vi "CV curve generator.vi"(0 "Lower bound (V)":dbl, 5 "Upper bound (V)":dbl, 7 "Start potential (V)":dbl, 9 "Stop potential (V)":dbl, 11 "Scan rate (mV/s)":dbl, 12 "Time (ms)":dbl, 13 "Number of cycles":u16) -> (4 "Actual potential":dbl, 15 "End":bool)   [LabVIEW 2015]
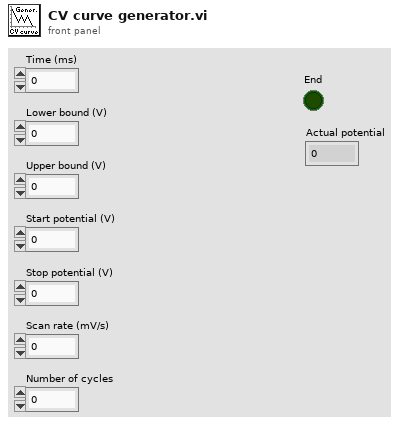
[diagram p1: front panel]
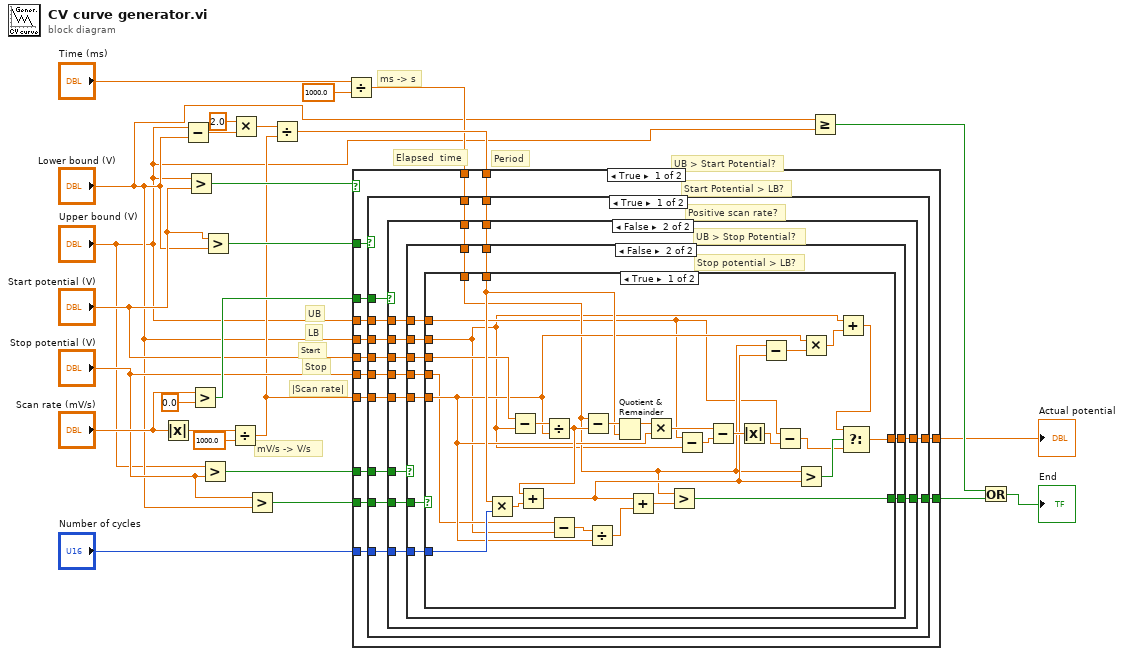
[diagram p0: block diagram]
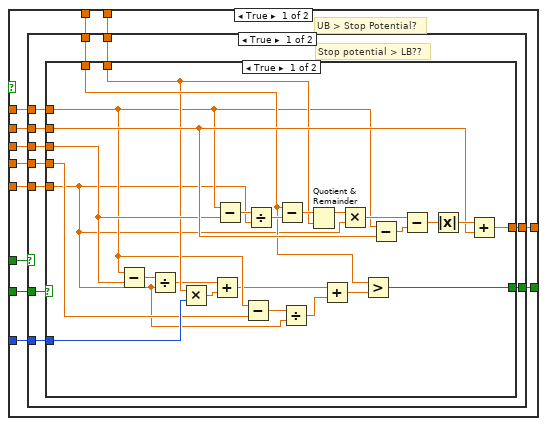
[diagram p2: hidden frame]
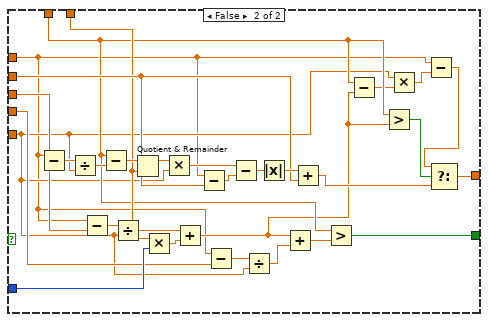
[diagram p3: hidden frame]
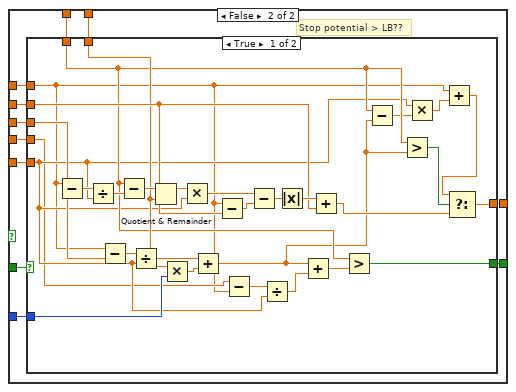
[diagram p4: hidden frame]
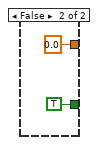
[diagram p5: hidden frame]
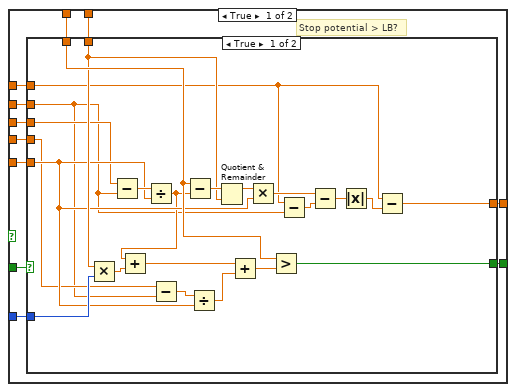
[diagram p6: hidden frame]
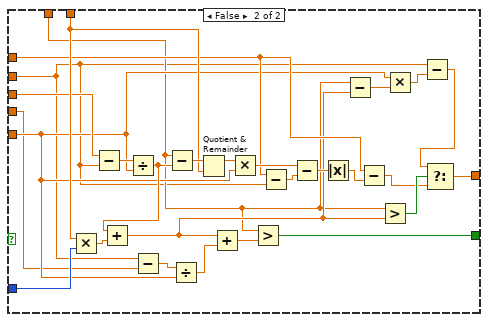
[diagram p7: hidden frame]
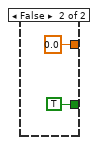
[diagram p8: hidden frame]
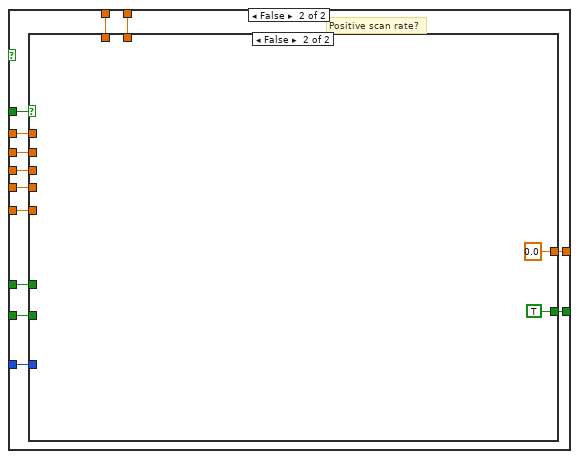
[diagram p9: hidden frame]
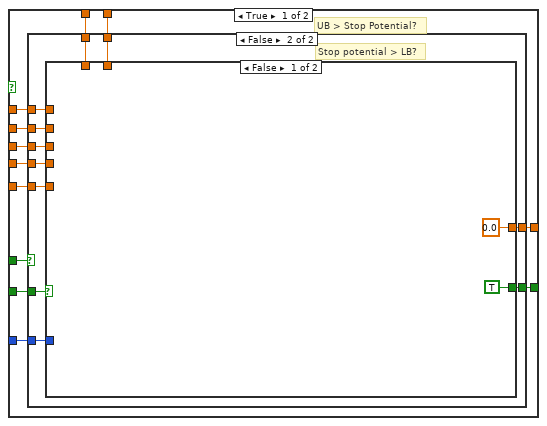
[diagram p10: hidden frame]
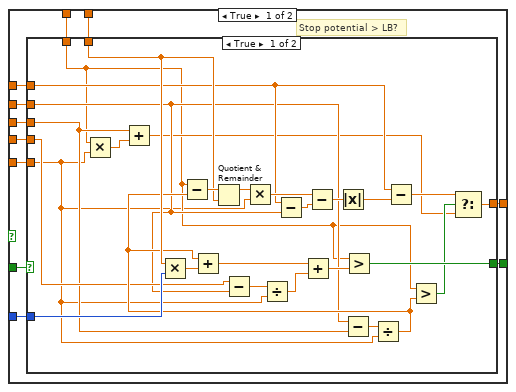
[diagram p11: hidden frame]
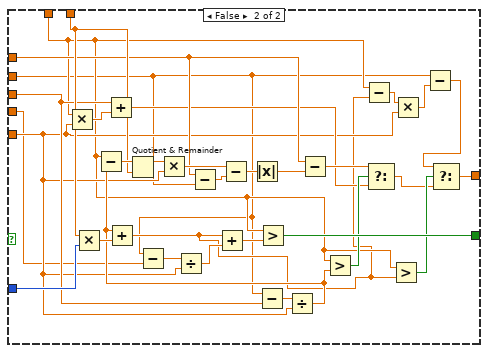
[diagram p12: hidden frame]
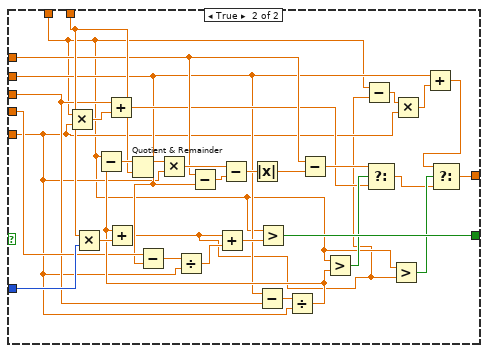
[diagram p13: hidden frame]
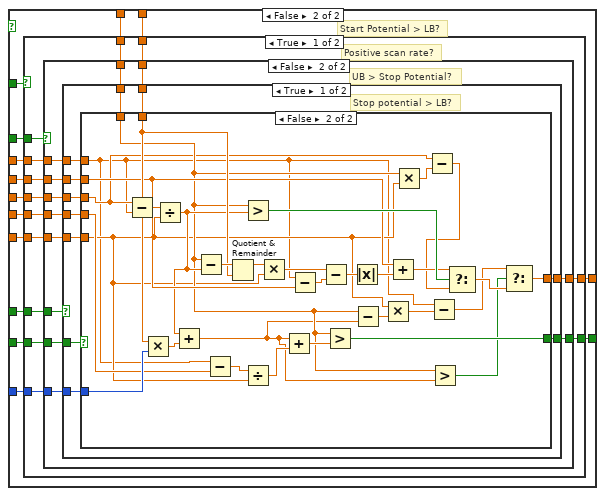
[diagram p14: hidden frame]
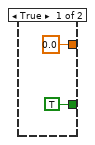
[diagram p15: hidden frame]
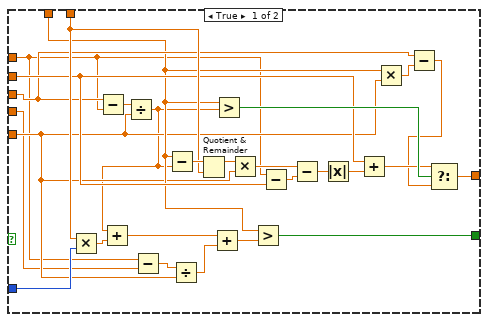
[diagram p16: hidden frame]
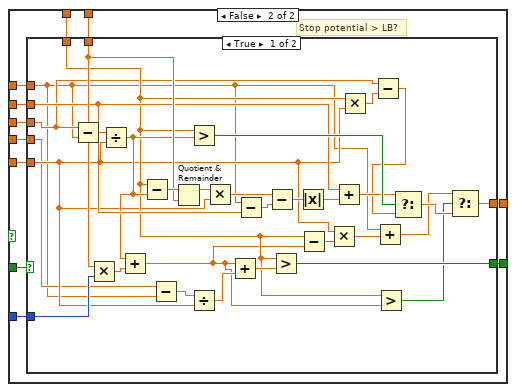
[diagram p17: hidden frame]
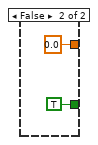
[diagram p18: hidden frame]
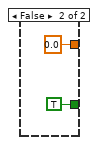
[diagram p19: hidden frame]
diagram:
  # "mV/s -> V/s"
  # "ms -> s"
  # "Elapsed  time"
  # "Period"
  # "|Scan rate|"
  # "Stop"
  # "Start"
  # "LB"
  # "UB"
  # "UB > Start Potential?"
  n1 = Absolute Value(x="Scan rate (mV/s)") -> (abs(x)=w17:dbl)
  n2 = Subtract(x="Upper bound (V)", y="Lower bound (V)") -> (x-y=w24:dbl)
  n3 = Greater?(x="Upper bound (V)", y="Start potential (V)") -> (0:w26:bool)
  n4 = Greater?(x="Scan rate (mV/s)", y=0.0) -> (0:w19:bool)
  n5 = Greater?(x="Upper bound (V)", y="Stop potential (V)") -> (0:w15:bool)
  n6 = Greater?(x="Start potential (V)", y="Lower bound (V)") -> (0:w25:bool)
  n7 = Divide(x=w17, y=1000.0) -> (x/y=w9:dbl)
  n8 = Multiply(x=2.0, y=w24) -> (x*y=w22:dbl)
  n9 = Greater?(x="Stop potential (V)", y="Lower bound (V)") -> (0:w14:bool)
  n10 = Divide(x=w22, y=w9) -> (x/y=w16:dbl)
  n11 = Divide(x="Time (ms)", y=1000.0) -> (x/y=w11:dbl)
  n12 = case shown="True" w26 {
    tunnel: w25 -> [w40 w445]
    tunnel: w19 -> [w39 w444]
    tunnel: "Upper bound (V)" -> [w38 w443]
    tunnel: "Lower bound (V)" -> [w37 w442]
    tunnel: "Start potential (V)" -> [w36 w441]
    tunnel: "Stop potential (V)" -> [w35 w440]
    tunnel: w9 -> [w34 w439]
    tunnel: w11 -> [w33 w438]
    tunnel: w16 -> [w32 w437]
    tunnel: [w31 w436] -> w2
    tunnel: w15 -> [w30 w435]
    tunnel: w14 -> [w29 w434]
    tunnel: [w28 w433] -> w7
    tunnel: "Number of cycles" -> [w27 w432]
    frame True {
      # "Start Potential > LB?"
      n13 = case shown="True" w40 {
        tunnel: w39 -> [w53 w302]
        tunnel: w38 -> [w52 w301]
        tunnel: w37 -> [w51 w300]
        tunnel: w36 -> [w50 w299]
        tunnel: w35 -> [w49 w298]
        tunnel: w34 -> [w48 w297]
        tunnel: w33 -> [w47 w296]
        tunnel: w32 -> [w46 w295]
        tunnel: [w45 w294] -> w31
        tunnel: w30 -> [w44 w293]
        tunnel: w29 -> [w43 w292]
        tunnel: [w42 w291] -> w28
        tunnel: w27 -> [w41 w290]
        frame True {
          # "Positive scan rate?"
          n14 = case shown="False" w53 {
            tunnel: w52 -> [w61 w182]
            tunnel: w51 -> [w60 w181]
            tunnel: w50 -> [w65 w186]
            tunnel: w49 -> [w54 w175]
            tunnel: w48 -> [w62 w183]
            tunnel: w47 -> [w64 w185]
            tunnel: w46 -> [w63 w184]
            tunnel: [w59 w180] -> w45
            tunnel: w44 -> [w58 w179]
            tunnel: w43 -> [w57 w178]
            tunnel: [w56 w177] -> w42
            tunnel: w41 -> [w55 w176]
            frame True {
              # "UB > Stop Potential?"
              n15 = case shown="True" w58 {
                tunnel: w65 -> [w76 w142]
                tunnel: w64 -> [w75 w141]
                tunnel: w63 -> [w74 w140]
                tunnel: w62 -> [w73 w139]
                tunnel: w61 -> [w72 w138]
                tunnel: w60 -> [w71 w137]
                tunnel: [w70 w136] -> w59
                tunnel: w57 -> [w69 w135]
                tunnel: [w68 w134] -> w56
                tunnel: w55 -> [w67 w133]
                tunnel: w54 -> [w66 w132]
                frame True {
                  # "Stop potential > LB??"
                  n16 = case shown="True" w69 {
                    tunnel: w76 -> [w89 w121]
                    tunnel: w75 -> [w90 w108]
                    tunnel: w74 -> [w87 w119]
                    tunnel: w73 -> [w77 w105]
                    tunnel: w72 -> [w83 w103]
                    tunnel: w71 -> [w93 w123]
                    tunnel: [w92 w111] -> w70
                    tunnel: [w91 w122] -> w68
                    tunnel: w67 -> [w86 w118]
                    tunnel: w66 -> [w82 w115]
                    frame True {
                      n17 = Subtract(x=w83, y=w89) -> (x-y=w88:dbl)
                      n18 = Divide(x=w88, y=w77) -> (x/y=w85:dbl)
                      n19 = Multiply(x=w87, y=w86) -> (x*y=w84:dbl)
                      n20 = Add(x=w85, y=w84) -> (x+y=w81:dbl)
                      n21 = Subtract(x=w83, y=w89) -> (x-y=w101:dbl)
                      n22 = Subtract(x=w83, y=w82) -> (x-y=w80:dbl)
                      n23 = Divide(x=w101, y=w77) -> (x/y=w100:dbl)
                      n24 = Subtract(x=w90, y=w100) -> (x-y=w99:dbl)
                      n25 = Divide(x=w80, y=w77) -> (x/y=w78:dbl)
                      n26 = Quotient & Remainder(x=w99, y=w87) -> (x-y*floor(x/y)=w98:dbl)  [unwired: 1 out]
                      n27 = Add(x=w81, y=w78) -> (x+y=w79:dbl)
                      n28 = Multiply(x=w98, y=w77) -> (x*y=w97:dbl)
                      n29 = Greater?(x=w90, y=w79) -> (0:w91:bool)
                      n30 = Subtract(x=w83, y=w93) -> (x-y=w96:dbl)
                      n31 = Subtract(x=w97, y=w96) -> (x-y=w95:dbl)
                      n32 = Absolute Value(x=w95) -> (abs(x)=w94:dbl)
                      n33 = Add(x=w94, y=w93) -> (x+y=w92:dbl)
                    }
                    frame False {
                      n34 = Subtract(x=w103, y=w121) -> (x-y=w131:dbl)
                      n35 = Divide(x=w131, y=w105) -> (x/y=w130:dbl)
                      n36 = Subtract(x=w103, y=w121) -> (x-y=w120:dbl)
                      n37 = Subtract(x=w108, y=w130) -> (x-y=w129:dbl)
                      n38 = Divide(x=w120, y=w105) -> (x/y=w117:dbl)
                      n39 = Quotient & Remainder(x=w129, y=w119) -> (x-y*floor(x/y)=w128:dbl)  [unwired: 1 out]
                      n40 = Multiply(x=w119, y=w118) -> (x*y=w116:dbl)
                      n41 = Multiply(x=w128, y=w105) -> (x*y=w127:dbl)
                      n42 = Add(x=w117, y=w116) -> (x+y=w107:dbl)
                      n43 = Subtract(x=w103, y=w123) -> (x-y=w126:dbl)
                      n44 = Subtract(x=w103, y=w115) -> (x-y=w114:dbl)
                      n45 = Subtract(x=w127, y=w126) -> (x-y=w125:dbl)
                      n46 = Divide(x=w114, y=w105) -> (x/y=w112:dbl)
                      n47 = Absolute Value(x=w125) -> (abs(x)=w124:dbl)
                      n48 = Add(x=w107, y=w112) -> (x+y=w113:dbl)
                      n49 = Add(x=w124, y=w123) -> (x+y=w110:dbl)
                      n50 = Greater?(x=w108, y=w113) -> (0:w122:bool)
                      n51 = Subtract(x=w108, y=w107) -> (x-y=w106:dbl)
                      n52 = Greater?(x=w108, y=w107) -> (0:w109:bool)
                      n53 = Multiply(x=w105, y=w106) -> (x*y=w104:dbl)
                      n54 = Subtract(x=w103, y=w104) -> (x-y=w102:dbl)
                      n55 = Select(t=w102, s=w109, f=w110) -> (s? t:f=w111:dbl)
                    }
                  }
                }
                frame False {
                  # "Stop potential > LB??"
                  n56 = case shown="True" w135 {
                    tunnel: w142 -> [w162 _]
                    tunnel: w141 -> [w150 _]
                    tunnel: w140 -> [w160 _]
                    tunnel: w139 -> [w147 _]
                    tunnel: w138 -> [w143 _]
                    tunnel: w137 -> [w164 _]
                    tunnel: [w153 0.0] -> w136
                    tunnel: [w163 TRUE] -> w134
                    tunnel: w133 -> [w159 _]
                    tunnel: w132 -> [w144 _]
                    frame True {
                      n57 = Subtract(x=w143, y=w162) -> (x-y=w172:dbl)
                      n58 = Divide(x=w172, y=w147) -> (x/y=w171:dbl)
                      n59 = Subtract(x=w143, y=w162) -> (x-y=w161:dbl)
                      n60 = Subtract(x=w150, y=w171) -> (x-y=w170:dbl)
                      n61 = Divide(x=w161, y=w147) -> (x/y=w158:dbl)
                      n62 = Quotient & Remainder(x=w170, y=w160) -> (x-y*floor(x/y)=w169:dbl)  [unwired: 1 out]
                      n63 = Multiply(x=w160, y=w159) -> (x*y=w157:dbl)
                      n64 = Multiply(x=w169, y=w147) -> (x*y=w168:dbl)
                      n65 = Add(x=w158, y=w157) -> (x+y=w149:dbl)
                      n66 = Subtract(x=w143, y=w164) -> (x-y=w167:dbl)
                      n67 = Subtract(x=w144, y=w143) -> (x-y=w156:dbl)
                      n68 = Subtract(x=w168, y=w167) -> (x-y=w166:dbl)
                      n69 = Divide(x=w156, y=w147) -> (x/y=w154:dbl)
                      n70 = Absolute Value(x=w166) -> (abs(x)=w165:dbl)
                      n71 = Add(x=w149, y=w154) -> (x+y=w155:dbl)
                      n72 = Add(x=w165, y=w164) -> (x+y=w152:dbl)
                      n73 = Greater?(x=w150, y=w155) -> (0:w163:bool)
                      n74 = Subtract(x=w150, y=w149) -> (x-y=w148:dbl)
                      n75 = Greater?(x=w150, y=w149) -> (0:w151:bool)
                      n76 = Multiply(x=w147, y=w148) -> (x*y=w146:dbl)
                      n77 = Add(x=w143, y=w146) -> (x+y=w145:dbl)
                      n78 = Select(t=w145, s=w151, f=w152) -> (s? t:f=w153:dbl)
                    }
                    frame False {
                    }
                  }
                }
              }
            }
            frame False {
              # "UB > Stop Potential?"
              n79 = case shown="False" w179 {
                tunnel: w186 -> [w197 w259]
                tunnel: w185 -> [w196 w258]
                tunnel: w184 -> [w195 w257]
                tunnel: w183 -> [w194 w256]
                tunnel: w182 -> [w193 w255]
                tunnel: w181 -> [w192 w254]
                tunnel: [w191 w253] -> w180
                tunnel: w178 -> [w190 w252]
                tunnel: [w189 w251] -> w177
                tunnel: w176 -> [w188 w250]
                tunnel: w175 -> [w187 w249]
                frame True {
                  # "Stop potential > LB?"
                  n80 = case shown="True" w190 {
                    tunnel: w197 -> [w203 w235]
                    tunnel: w196 -> [w212 w223]
                    tunnel: w195 -> [w211 w241]
                    tunnel: w194 -> [w204 w225]
                    tunnel: w193 -> [w201 w233]
                    tunnel: w192 -> [w198 w222]
                    tunnel: [w214 w226] -> w191
                    tunnel: [w213 w242] -> w189
                    tunnel: w188 -> [w210 w240]
                    tunnel: w187 -> [w199 w221]
                    frame True {
                      n81 = Multiply(x=w211, y=w210) -> (x*y=w209:dbl)
                      n82 = Subtract(x=w203, y=w198) -> (x-y=w220:dbl)
                      n83 = Divide(x=w220, y=w204) -> (x/y=w200:dbl)
                      n84 = Add(x=w200, y=w209) -> (x+y=w208:dbl)
                      n85 = Subtract(x=w199, y=w198) -> (x-y=w207:dbl)
                      n86 = Subtract(x=w212, y=w200) -> (x-y=w219:dbl)
                      n87 = Divide(x=w207, y=w204) -> (x/y=w205:dbl)
                      n88 = Quotient & Remainder(x=w219, y=w211) -> (x-y*floor(x/y)=w218:dbl)  [unwired: 1 out]
                      n89 = Add(x=w208, y=w205) -> (x+y=w206:dbl)
                      n90 = Multiply(x=w218, y=w204) -> (x*y=w217:dbl)
                      n91 = Greater?(x=w212, y=w206) -> (0:w213:bool)
                      n92 = Subtract(x=w201, y=w198) -> (x-y=w216:dbl)
                      n93 = Subtract(x=w217, y=w216) -> (x-y=w215:dbl)
                      n94 = Absolute Value(x=w215) -> (abs(x)=w202:dbl)
                      n95 = Subtract(x=w201, y=w202) -> (x-y=w214:dbl)
                    }
                    frame False {
                      n96 = Multiply(x=w241, y=w240) -> (x*y=w239:dbl)
                      n97 = Subtract(x=w235, y=w222) -> (x-y=w248:dbl)
                      n98 = Divide(x=w248, y=w225) -> (x/y=w232:dbl)
                      n99 = Add(x=w232, y=w239) -> (x+y=w224:dbl)
                      n100 = Subtract(x=w222, y=w221) -> (x-y=w238:dbl)
                      n101 = Subtract(x=w223, y=w232) -> (x-y=w247:dbl)
                      n102 = Divide(x=w238, y=w225) -> (x/y=w236:dbl)
                      n103 = Quotient & Remainder(x=w247, y=w241) -> (x-y*floor(x/y)=w246:dbl)  [unwired: 1 out]
                      n104 = Add(x=w224, y=w236) -> (x+y=w237:dbl)
                      n105 = Multiply(x=w246, y=w225) -> (x*y=w245:dbl)
                      n106 = Greater?(x=w223, y=w237) -> (0:w242:bool)
                      n107 = Subtract(x=w233, y=w222) -> (x-y=w244:dbl)
                      n108 = Subtract(x=w245, y=w244) -> (x-y=w243:dbl)
                      n109 = Absolute Value(x=w243) -> (abs(x)=w234:dbl)
                      n110 = Subtract(x=w223, y=w224) -> (x-y=w229:dbl)
                      n111 = Subtract(x=w233, y=w234) -> (x-y=w227:dbl)
                      n112 = Greater?(x=w223, y=w224) -> (0:w228:bool)
                      n113 = Multiply(x=w225, y=w229) -> (x*y=w230:dbl)
                      n114 = Subtract(x=w222, y=w230) -> (x-y=w231:dbl)
                      n115 = Select(t=w231, s=w228, f=w227) -> (s? t:f=w226:dbl)
                    }
                  }
                }
                frame False {
                  # "Stop potential > LB?"
                  n116 = case shown="True" w252 {
                    tunnel: w259 -> [w274 _]
                    tunnel: w258 -> [w263 _]
                    tunnel: w257 -> [w280 _]
                    tunnel: w256 -> [w265 _]
                    tunnel: w255 -> [w261 _]
                    tunnel: w254 -> [w260 _]
                    tunnel: [w266 0.0] -> w253
                    tunnel: [w281 TRUE] -> w251
                    tunnel: w250 -> [w279 _]
                    tunnel: w249 -> [w262 _]
                    frame True {
                      n117 = Multiply(x=w280, y=w279) -> (x*y=w278:dbl)
                      n118 = Subtract(x=w274, y=w260) -> (x-y=w287:dbl)
                      n119 = Divide(x=w287, y=w265) -> (x/y=w272:dbl)
                      n120 = Add(x=w272, y=w278) -> (x+y=w264:dbl)
                      n121 = Subtract(x=w262, y=w260) -> (x-y=w277:dbl)
                      n122 = Subtract(x=w263, y=w272) -> (x-y=w286:dbl)
                      n123 = Divide(x=w277, y=w265) -> (x/y=w275:dbl)
                      n124 = Quotient & Remainder(x=w286, y=w280) -> (x-y*floor(x/y)=w285:dbl)  [unwired: 1 out]
                      n125 = Add(x=w264, y=w275) -> (x+y=w276:dbl)
                      n126 = Multiply(x=w285, y=w265) -> (x*y=w284:dbl)
                      n127 = Greater?(x=w263, y=w276) -> (0:w281:bool)
                      n128 = Subtract(x=w261, y=w260) -> (x-y=w283:dbl)
                      n129 = Subtract(x=w284, y=w283) -> (x-y=w282:dbl)
                      n130 = Absolute Value(x=w282) -> (abs(x)=w273:dbl)
                      n131 = Subtract(x=w263, y=w264) -> (x-y=w269:dbl)
                      n132 = Subtract(x=w261, y=w273) -> (x-y=w267:dbl)
                      n133 = Greater?(x=w263, y=w264) -> (0:w268:bool)
                      n134 = Multiply(x=w265, y=w269) -> (x*y=w270:dbl)
                      n135 = Add(x=w260, y=w270) -> (x+y=w271:dbl)
                      n136 = Select(t=w271, s=w268, f=w267) -> (s? t:f=w266:dbl)
                    }
                    frame False {
                    }
                  }
                }
              }
            }
          }
        }
        frame False {
          # "Positive scan rate?"
          n137 = case shown="False" w302 {
            tunnel: w301 -> [w310 _]
            tunnel: w300 -> [w309 _]
            tunnel: w299 -> [w314 _]
            tunnel: w298 -> [w303 _]
            tunnel: w297 -> [w311 _]
            tunnel: w296 -> [w313 _]
            tunnel: w295 -> [w312 _]
            tunnel: [w308 0.0] -> w294
            tunnel: w293 -> [w307 _]
            tunnel: w292 -> [w306 _]
            tunnel: [w305 TRUE] -> w291
            tunnel: w290 -> [w304 _]
            frame True {
              # "UB > Stop Potential?"
              n138 = case shown="False" w307 {
                tunnel: w314 -> [w325 w395]
                tunnel: w313 -> [w324 w394]
                tunnel: w312 -> [w323 w393]
                tunnel: w311 -> [w322 w392]
                tunnel: w310 -> [w321 w391]
                tunnel: w309 -> [w320 w390]
                tunnel: [w319 w389] -> w308
                tunnel: w306 -> [w318 w388]
                tunnel: [w317 w387] -> w305
                tunnel: w304 -> [w316 w386]
                tunnel: w303 -> [w315 w385]
                frame True {
                  # "Stop potential > LB?"
                  n139 = case shown="True" w318 {
                    tunnel: w325 -> [w329 w365]
                    tunnel: w324 -> [w327 w356]
                    tunnel: w323 -> [w346 w378]
                    tunnel: w322 -> [w326 w358]
                    tunnel: w321 -> [w334 w368]
                    tunnel: w320 -> [w331 w353]
                    tunnel: [w338 w363] -> w319
                    tunnel: [w347 w379] -> w317
                    tunnel: w316 -> [w345 w377]
                    tunnel: w315 -> [w332 w354]
                    frame True {
                      n140 = Multiply(x=w327, y=w326) -> (x*y=w330:dbl)
                      n141 = Add(x=w329, y=w330) -> (x+y=w328:dbl)
                      n142 = Multiply(x=w346, y=w345) -> (x*y=w344:dbl)
                      n143 = Subtract(x=w332, y=w331) -> (x-y=w342:dbl)
                      n144 = Divide(x=w342, y=w326) -> (x/y=w340:dbl)
                      n145 = Subtract(x=w334, y=w331) -> (x-y=w349:dbl)
                      n146 = Subtract(x=w331, y=w329) -> (x-y=w339:dbl)
                      n147 = Divide(x=w339, y=w326) -> (x/y=w333:dbl)
                      n148 = Subtract(x=w327, y=w333) -> (x-y=w352:dbl)
                      n149 = Add(x=w333, y=w344) -> (x+y=w343:dbl)
                      n150 = Quotient & Remainder(x=w352, y=w346) -> (x-y*floor(x/y)=w351:dbl)  [unwired: 1 out]
                      n151 = Multiply(x=w351, y=w326) -> (x*y=w350:dbl)
                      n152 = Add(x=w343, y=w340) -> (x+y=w341:dbl)
                      n153 = Subtract(x=w350, y=w349) -> (x-y=w348:dbl)
                      n154 = Absolute Value(x=w348) -> (abs(x)=w335:dbl)
                      n155 = Greater?(x=w327, y=w341) -> (0:w347:bool)
                      n156 = Subtract(x=w334, y=w335) -> (x-y=w336:dbl)
                      n157 = Greater?(x=w327, y=w333) -> (0:w337:bool)
                      n158 = Select(t=w336, s=w337, f=w328) -> (s? t:f=w338:dbl)
                    }
                    frame False {
                      n159 = Multiply(x=w356, y=w358) -> (x*y=w366:dbl)
                      n160 = Multiply(x=w378, y=w377) -> (x*y=w376:dbl)
                      n161 = Add(x=w365, y=w366) -> (x+y=w364:dbl)
                      n162 = Subtract(x=w353, y=w354) -> (x-y=w375:dbl)
                      n163 = Divide(x=w375, y=w358) -> (x/y=w373:dbl)
                      n164 = Subtract(x=w368, y=w353) -> (x-y=w381:dbl)
                      n165 = Subtract(x=w353, y=w365) -> (x-y=w372:dbl)
                      n166 = Divide(x=w372, y=w358) -> (x/y=w367:dbl)
                      n167 = Subtract(x=w356, y=w367) -> (x-y=w384:dbl)
                      n168 = Add(x=w367, y=w376) -> (x+y=w355:dbl)
                      n169 = Quotient & Remainder(x=w384, y=w378) -> (x-y*floor(x/y)=w383:dbl)  [unwired: 1 out]
                      n170 = Multiply(x=w383, y=w358) -> (x*y=w382:dbl)
                      n171 = Add(x=w355, y=w373) -> (x+y=w374:dbl)
                      n172 = Subtract(x=w382, y=w381) -> (x-y=w380:dbl)
                      n173 = Absolute Value(x=w380) -> (abs(x)=w369:dbl)
                      n174 = Greater?(x=w356, y=w374) -> (0:w379:bool)
                      n175 = Subtract(x=w368, y=w369) -> (x-y=w370:dbl)
                      n176 = Greater?(x=w356, y=w367) -> (0:w371:bool)
                      n177 = Subtract(x=w356, y=w355) -> (x-y=w357:dbl)
                      n178 = Select(t=w370, s=w371, f=w364) -> (s? t:f=w361:dbl)
                      n179 = Greater?(x=w356, y=w355) -> (0:w362:bool)
                      n180 = Multiply(x=w357, y=w358) -> (x*y=w359:dbl)
                      n181 = Subtract(x=w353, y=w359) -> (x-y=w360:dbl)
                      n182 = Select(t=w360, s=w362, f=w361) -> (s? t:f=w363:dbl)
                    }
                  }
                }
                frame False {
                  # "Stop potential > LB?"
                  n183 = case shown="False" w388 {
                    tunnel: w395 -> [_ w409]
                    tunnel: w394 -> [_ w399]
                    tunnel: w393 -> [_ w423]
                    tunnel: w392 -> [_ w401]
                    tunnel: w391 -> [_ w413]
                    tunnel: w390 -> [_ w404]
                    tunnel: [0.0 w407] -> w389
                    tunnel: [TRUE w424] -> w387
                    tunnel: w386 -> [_ w422]
                    tunnel: w385 -> [_ w411]
                    frame False {
                    }
                    frame True {
                      n184 = Multiply(x=w399, y=w401) -> (x*y=w410:dbl)
                      n185 = Multiply(x=w423, y=w422) -> (x*y=w421:dbl)
                      n186 = Add(x=w409, y=w410) -> (x+y=w408:dbl)
                      n187 = Subtract(x=w411, y=w404) -> (x-y=w420:dbl)
                      n188 = Divide(x=w420, y=w401) -> (x/y=w418:dbl)
                      n189 = Subtract(x=w413, y=w404) -> (x-y=w426:dbl)
                      n190 = Subtract(x=w404, y=w409) -> (x-y=w417:dbl)
                      n191 = Divide(x=w417, y=w401) -> (x/y=w412:dbl)
                      n192 = Subtract(x=w399, y=w412) -> (x-y=w429:dbl)
                      n193 = Add(x=w412, y=w421) -> (x+y=w398:dbl)
                      n194 = Quotient & Remainder(x=w429, y=w423) -> (x-y*floor(x/y)=w428:dbl)  [unwired: 1 out]
                      n195 = Multiply(x=w428, y=w401) -> (x*y=w427:dbl)
                      n196 = Add(x=w398, y=w418) -> (x+y=w419:dbl)
                      n197 = Subtract(x=w427, y=w426) -> (x-y=w425:dbl)
                      n198 = Absolute Value(x=w425) -> (abs(x)=w414:dbl)
                      n199 = Greater?(x=w399, y=w419) -> (0:w424:bool)
                      n200 = Subtract(x=w413, y=w414) -> (x-y=w415:dbl)
                      n201 = Greater?(x=w399, y=w412) -> (0:w416:bool)
                      n202 = Subtract(x=w399, y=w398) -> (x-y=w400:dbl)
                      n203 = Select(t=w415, s=w416, f=w408) -> (s? t:f=w405:dbl)
                      n204 = Greater?(x=w399, y=w398) -> (0:w406:bool)
                      n205 = Multiply(x=w400, y=w401) -> (x*y=w402:dbl)
                      n206 = Add(x=w404, y=w402) -> (x+y=w403:dbl)
                      n207 = Select(t=w403, s=w406, f=w405) -> (s? t:f=w407:dbl)
                    }
                  }
                }
              }
            }
            frame False {
            }
          }
        }
      }
    }
    frame False {
      # "Start Potential > LB?"
      n208 = case shown="True" w445 {
        tunnel: w444 -> [w458 _]
        tunnel: w443 -> [w457 _]
        tunnel: w442 -> [w456 _]
        tunnel: w441 -> [w455 _]
        tunnel: w440 -> [w454 _]
        tunnel: w439 -> [w453 _]
        tunnel: w438 -> [w452 _]
        tunnel: w437 -> [w451 _]
        tunnel: [w450 0.0] -> w436
        tunnel: w435 -> [w449 _]
        tunnel: w434 -> [w448 _]
        tunnel: [w447 TRUE] -> w433
        tunnel: w432 -> [w446 _]
        frame True {
          # "Positive scan rate?"
          n209 = case shown="False" w458 {
            tunnel: w457 -> [_ w468]
            tunnel: w456 -> [_ w467]
            tunnel: w455 -> [_ w472]
            tunnel: w454 -> [_ w461]
            tunnel: w453 -> [_ w469]
            tunnel: w452 -> [_ w471]
            tunnel: w451 -> [_ w470]
            tunnel: [0.0 w466] -> w450
            tunnel: w449 -> [_ w465]
            tunnel: w448 -> [_ w464]
            tunnel: [TRUE w463] -> w447
            tunnel: w446 -> [_ w462]
            frame True {
            }
            frame False {
              # "UB > Stop Potential?"
              n210 = case shown="True" w465 {
                tunnel: w472 -> [w483 w553]
                tunnel: w471 -> [w482 w552]
                tunnel: w470 -> [w481 w551]
                tunnel: w469 -> [w480 w550]
                tunnel: w468 -> [w479 w549]
                tunnel: w467 -> [w478 w548]
                tunnel: [w477 w547] -> w466
                tunnel: w464 -> [w476 w546]
                tunnel: [w475 w545] -> w463
                tunnel: w462 -> [w474 w544]
                tunnel: w461 -> [w473 w543]
                frame True {
                  # "Stop potential > LB?"
                  n211 = case shown="False" w476 {
                    tunnel: w483 -> [w490 w513]
                    tunnel: w482 -> [w489 w518]
                    tunnel: w481 -> [w504 w536]
                    tunnel: w480 -> [w488 w515]
                    tunnel: w479 -> [w485 w511]
                    tunnel: w478 -> [w492 w526]
                    tunnel: [w496 w521] -> w477
                    tunnel: [w505 w537] -> w475
                    tunnel: w474 -> [w503 w535]
                    tunnel: w473 -> [w484 w522]
                    frame True {
                      n212 = Multiply(x=w504, y=w503) -> (x*y=w502:dbl)
                      n213 = Subtract(x=w490, y=w485) -> (x-y=w495:dbl)
                      n214 = Divide(x=w495, y=w488) -> (x/y=w486:dbl)
                      n215 = Add(x=w486, y=w502) -> (x+y=w501:dbl)
                      n216 = Subtract(x=w485, y=w484) -> (x-y=w500:dbl)
                      n217 = Subtract(x=w489, y=w486) -> (x-y=w510:dbl)
                      n218 = Divide(x=w500, y=w488) -> (x/y=w498:dbl)
                      n219 = Quotient & Remainder(x=w510, y=w504) -> (x-y*floor(x/y)=w509:dbl)  [unwired: 1 out]
                      n220 = Add(x=w501, y=w498) -> (x+y=w499:dbl)
                      n221 = Greater?(x=w489, y=w486) -> (0:w494:bool)
                      n222 = Multiply(x=w509, y=w488) -> (x*y=w508:dbl)
                      n223 = Greater?(x=w489, y=w499) -> (0:w505:bool)
                      n224 = Subtract(x=w485, y=w492) -> (x-y=w507:dbl)
                      n225 = Subtract(x=w508, y=w507) -> (x-y=w506:dbl)
                      n226 = Absolute Value(x=w506) -> (abs(x)=w497:dbl)
                      n227 = Add(x=w492, y=w497) -> (x+y=w493:dbl)
                      n228 = Multiply(x=w489, y=w488) -> (x*y=w491:dbl)
                      n229 = Subtract(x=w490, y=w491) -> (x-y=w487:dbl)
                      n230 = Select(t=w493, s=w494, f=w487) -> (s? t:f=w496:dbl)
                    }
                    frame False {
                      n231 = Subtract(x=w513, y=w511) -> (x-y=w529:dbl)
                      n232 = Multiply(x=w536, y=w535) -> (x*y=w534:dbl)
                      n233 = Divide(x=w529, y=w515) -> (x/y=w523:dbl)
                      n234 = Add(x=w523, y=w534) -> (x+y=w517:dbl)
                      n235 = Subtract(x=w518, y=w523) -> (x-y=w542:dbl)
                      n236 = Subtract(x=w511, y=w522) -> (x-y=w533:dbl)
                      n237 = Quotient & Remainder(x=w542, y=w536) -> (x-y*floor(x/y)=w541:dbl)  [unwired: 1 out]
                      n238 = Greater?(x=w518, y=w523) -> (0:w528:bool)
                      n239 = Divide(x=w533, y=w515) -> (x/y=w531:dbl)
                      n240 = Multiply(x=w541, y=w515) -> (x*y=w540:dbl)
                      n241 = Add(x=w517, y=w531) -> (x+y=w532:dbl)
                      n242 = Subtract(x=w511, y=w526) -> (x-y=w539:dbl)
                      n243 = Subtract(x=w540, y=w539) -> (x-y=w538:dbl)
                      n244 = Greater?(x=w518, y=w532) -> (0:w537:bool)
                      n245 = Absolute Value(x=w538) -> (abs(x)=w530:dbl)
                      n246 = Subtract(x=w518, y=w517) -> (x-y=w516:dbl)
                      n247 = Multiply(x=w515, y=w516) -> (x*y=w514:dbl)
                      n248 = Add(x=w526, y=w530) -> (x+y=w527:dbl)
                      n249 = Multiply(x=w518, y=w515) -> (x*y=w525:dbl)
                      n250 = Subtract(x=w513, y=w525) -> (x-y=w524:dbl)
                      n251 = Subtract(x=w511, y=w514) -> (x-y=w512:dbl)
                      n252 = Greater?(x=w518, y=w517) -> (0:w519:bool)
                      n253 = Select(t=w527, s=w528, f=w524) -> (s? t:f=w520:dbl)
                      n254 = Select(t=w512, s=w519, f=w520) -> (s? t:f=w521:dbl)
                    }
                  }
                }
                frame False {
                  # "Stop potential > LB?"
                  n255 = case shown="True" w546 {
                    tunnel: w553 -> [w557 _]
                    tunnel: w552 -> [w562 _]
                    tunnel: w551 -> [w579 _]
                    tunnel: w550 -> [w559 _]
                    tunnel: w549 -> [w554 _]
                    tunnel: w548 -> [w569 _]
                    tunnel: [w565 0.0] -> w547
                    tunnel: [w580 TRUE] -> w545
                    tunnel: w544 -> [w578 _]
                    tunnel: w543 -> [w555 _]
                    frame True {
                      n256 = Subtract(x=w557, y=w554) -> (x-y=w572:dbl)
                      n257 = Multiply(x=w579, y=w578) -> (x*y=w577:dbl)
                      n258 = Divide(x=w572, y=w559) -> (x/y=w566:dbl)
                      n259 = Add(x=w566, y=w577) -> (x+y=w561:dbl)
                      n260 = Subtract(x=w562, y=w566) -> (x-y=w585:dbl)
                      n261 = Subtract(x=w555, y=w554) -> (x-y=w576:dbl)
                      n262 = Quotient & Remainder(x=w585, y=w579) -> (x-y*floor(x/y)=w584:dbl)  [unwired: 1 out]
                      n263 = Greater?(x=w562, y=w566) -> (0:w571:bool)
                      n264 = Divide(x=w576, y=w559) -> (x/y=w574:dbl)
                      n265 = Multiply(x=w584, y=w559) -> (x*y=w583:dbl)
                      n266 = Add(x=w561, y=w574) -> (x+y=w575:dbl)
                      n267 = Subtract(x=w554, y=w569) -> (x-y=w582:dbl)
                      n268 = Subtract(x=w583, y=w582) -> (x-y=w581:dbl)
                      n269 = Greater?(x=w562, y=w575) -> (0:w580:bool)
                      n270 = Absolute Value(x=w581) -> (abs(x)=w573:dbl)
                      n271 = Subtract(x=w562, y=w561) -> (x-y=w560:dbl)
                      n272 = Multiply(x=w559, y=w560) -> (x*y=w558:dbl)
                      n273 = Add(x=w569, y=w573) -> (x+y=w570:dbl)
                      n274 = Multiply(x=w562, y=w559) -> (x*y=w568:dbl)
                      n275 = Subtract(x=w557, y=w568) -> (x-y=w567:dbl)
                      n276 = Add(x=w554, y=w558) -> (x+y=w556:dbl)
                      n277 = Greater?(x=w562, y=w561) -> (0:w563:bool)
                      n278 = Select(t=w570, s=w571, f=w567) -> (s? t:f=w564:dbl)
                      n279 = Select(t=w556, s=w563, f=w564) -> (s? t:f=w565:dbl)
                    }
                    frame False {
                    }
                  }
                }
              }
            }
          }
        }
        frame False {
        }
      }
    }
  }
  "Actual potential" <- w2
  n280 = Greater Or Equal?(x="Lower bound (V)", y="Upper bound (V)") -> (x >= y?=w6:bool)
  n281 = Or(x=w6, y=w7) -> (x .or. y?=→"End":bool)
